vi "FRCts20_Backend_EventRoot_PPD_return.vi"(7 "Events":T1, 8 "error in (no error)":errorcluster, 10 "rows affected":i32) -> (0 "error out":errorcluster, 3 "data string":string)   [LabVIEW 2013, in "FRCts20_Backend_Engine.lvlib"]
doc: "Returns whether a new event was successfully created"
uses:
  FRCts20_Backend_Engine.lvlib
  FRCts20_Backend_API/FRCts20_Backend_API_EventRoot.ctl
  FRCts20_Backend_API/FRCts20_Backend_API.lvlib
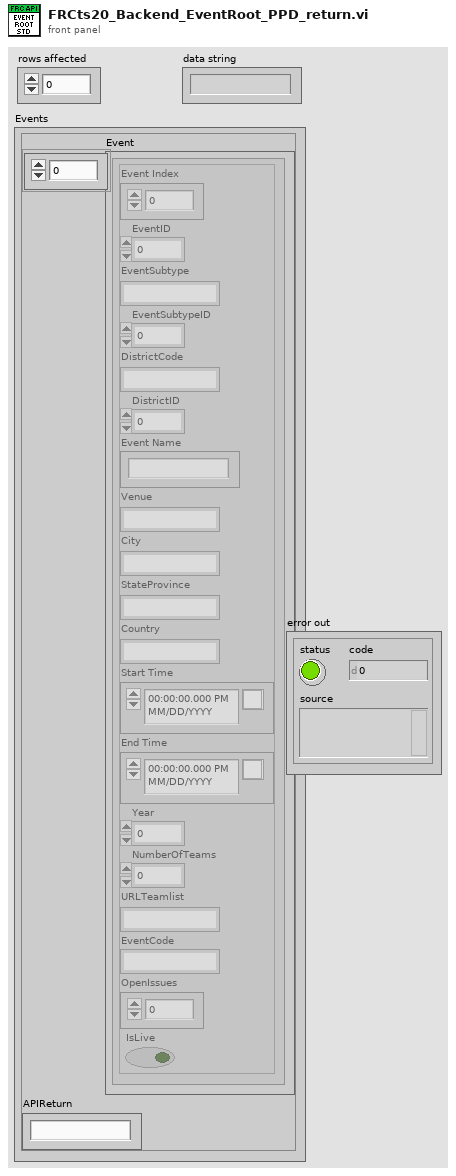
[diagram p1: front panel]
types:
  T1 = typedef "FRCts20_Backend_API.lvlib/FRCts20_Backend_API_EventRoot.ctl" = cluster{"Event":cluster{"Event Index":u32, "EventID":u32, "EventSubtype":string, "EventSubtypeID":u32, "DistrictCode":string, "DistrictID":u32, "Event Name":string, "Venue":string, "City":string, "StateProvince":string, "Country":string, "Start Time":timestamp, "End Time":timestamp, "Year":u32, "NumberOfTeams":u32, "URLTeamlist":string, "EventCode":string, "OpenIssues":u8, "IsLive":bool}[], "APIReturn":string}
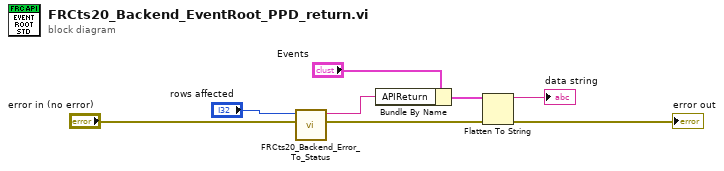
[diagram p0: block diagram]
diagram:
  n1 = call "FRCts20_Backend_Error_To_Status.vi"("error in (no error)"="error in (no error)", "rows affected"="rows affected") -> ("error out"=w4:errorcluster, "String"=w5:string)  [unwired: 8 in]
  n2 = Bundle By Name(cluster="Events", "APIReturn"=w5) -> (w3:T1)
  n3 = Flatten To String(anything=w3, error in (no error)=w4) -> (data string=→"data string":string, error out=→"error out":errorcluster)  [unwired: 2 in, 1 out]
